vi "Launch_browser.vi"(5 "path":string="WebConfig/index.php", 6 "error in":errorcluster, 9 "host address":string="192.168.1.34") -> (0 "error out":errorcluster, 3 "URL out":string="192.168.1.34")   [LabVIEW 2014, in "Raspberry Pi Compatible Compiler for LabVIEW.lvlib" / "Autodetect.lvlib"]
doc: "Builds a URL from an IP address and the default home path then launches the default browser with that location."
uses:
  Autodetect.lvlib
  <vilib>/Platform/browser.llb/Open URL in Default Browser (string).vi
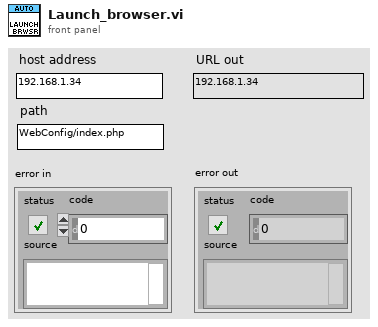
[diagram p1: front panel]
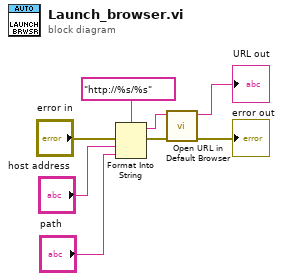
[diagram p0: block diagram]
diagram:
  n1 = Format Into String(format string="http://%s/%s", error in="error in", "host address", "path") -> (resulting string=w5:string, error out=w4:errorcluster)  [unwired: 1 in]
  n2 = call-poly <vilib>:"Open URL in Default Browser.vi"("error in (no error)"=w4, "URL"=w5) -> ("error out"=→"error out":errorcluster, "URL out"=→"URL out":string)  [unwired: 4 in]
